vi "VDH-RequestCalibration.vi"(8 "error in (no error)":errorcluster, 10 "Calibration Type":T1=enum."Short", 11 "VDH-VNA_data_handler in":refnum<class "VDH-VNA_data_handler.lvclass">) -> (0 "error out":errorcluster, 3 "VDH-VNA_data_handler out":refnum<class "VDH-VNA_data_handler.lvclass">)   [LabVIEW 2020, in "VDH-VNA_data_handler.lvlib" / "VDH-VNA_data_handler.lvclass"]
uses:
  VDH-VNA_data_handler.lvclass
  VDH-Calibration_enum.ctl
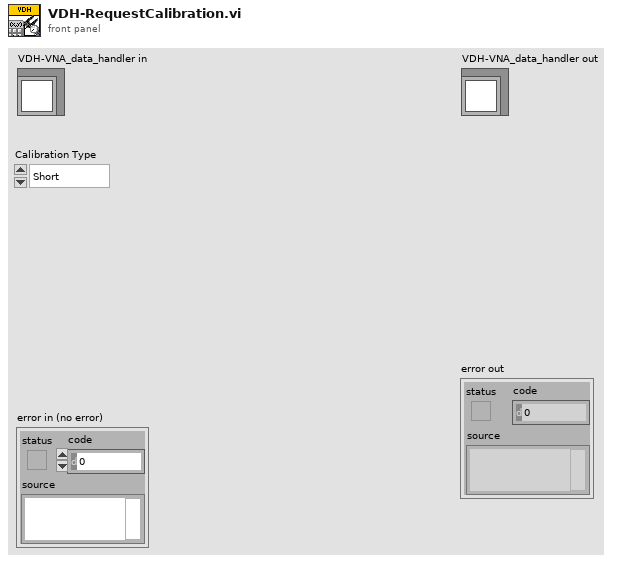
[diagram p1: front panel]
types:
  T1 = typedef "VDH-VNA_data_handler.lvlib/VDH-VNA_data_handler.lvclass/VDH-Calibration_enum.ctl" = enum16{"Non", "Short", "Open", "Load", "Through", "Permativity"}
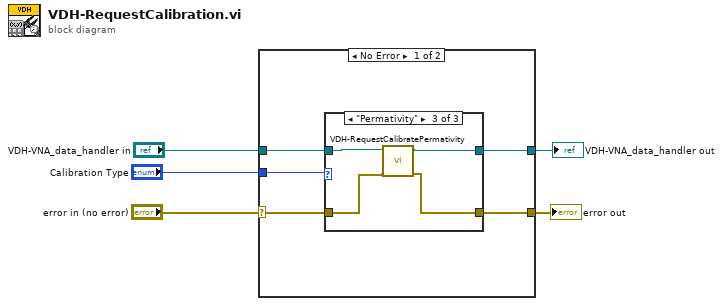
[diagram p0: block diagram]
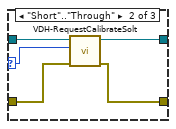
[diagram p3: hidden frame]
diagram:
  n1 = case shown="No Error" "error in (no error)" {
    selector: "error in (no error)" -> [w9 w23]
    tunnel: [w6 w23] -> w4
    tunnel: [w7 w22] -> w2
    tunnel: "VDH-VNA_data_handler in" -> [w8 w22]
    tunnel: "Calibration Type" -> [w10 _]
    frame No Error {
      n2 = case shown="\"Permativity\"" w10 {
        selector: w10 -> [_ w14 _]
        tunnel: w9 -> [w11 w16 w21]
        tunnel: w8 -> [w12 w17 w20]
        tunnel: [w12 w15 w19] -> w7
        tunnel: [w11 w13 w18] -> w6
        frame "Non", Default {
        }
        frame "Short".."Through" {
          n3 = call "VDH-RequestCalibrateSolt.vi"("error in (no error)"=w16, "SOLT"=w14, "VDH-VNA_data_handler in"=w17) -> ("error out"=w13:errorcluster, "VDH-VNA_data_handler out"=w15:refnum<class "VDH-VNA_data_handler.lvclass">)  [unwired: 7 in]
        }
        frame "Permativity" {
          n4 = call "VDH-RequestCalibratePermativity.vi"("error in (no error)"=w21, "VDH-VNA_data_handler in"=w20) -> ("error out"=w18:errorcluster, "VDH-VNA_data_handler out"=w19:refnum<class "VDH-VNA_data_handler.lvclass">)  [unwired: 8 in]
        }
      }
    }
    frame Error {
    }
  }
  "error out" <- w4
  "VDH-VNA_data_handler out" <- w2
